vi "Read Spectra from Data Object.vi"(8 "error in (no error)":errorcluster, 10 "component":T1=32 items=["Magnitude^2"=37, "Magnitude"=32, "Phase"=33, "Real"=34, "Imaginary"=35, "Coherence"=36, "Unknown"=99], 11 "Y (1 Ch) in":refnum<class "Y (1 Ch).lvclass">) -> (0 "error out":errorcluster, 1 "spectra info":T2[](array[typedef]) {"x-axis units" items=["Time (s)"=0, "Frequency-CB (Hz)"=1, "Frequency-CPB (Hz)"=1248, "Frequency-Arbitrary (Hz)"=2357, "Quefrency (s)"=2, "Revolutions (rev)"=3, "Order"=4, "Speed (RPM)"=11, "Speed (rad/s)"=21, "Index"=65535]; "weighting filter" items=["Linear", "A-weighting", "B-weighting", "C-weighting", "ITU-R 468-4", "Dolby", "CCITT", "C-message", "Wb", "Wc", "Wd", "We", "Wf", "Wh", "Wj", "Wk", "Wm", "AES17 20 kHz lowpass", "AES17 40 kHz lowpass", "AES17 20 kHz highpass", "AES17 40 kHz highpass"]; "dB reference [EU]" format="%.2f"; "engineering units" items=["custom..."=0, "V"=1, "A"=21, "C"=30, "pC"=31, "s"=32, "-"=29, "Pa"=2, "N"=20, "g"=3, "m/s^2"=4, "m/s"=5, "m"=6, "mm/s"=12, "mm"=13, "micron/s"=14, "micron"=15, "in/s^2"=7, "in/s"=8, "in"=9, "mil/s"=10, "mil"=11, "rad/s^2"=16, "rad/s"=17, "rad"=18, "deg/s^2"=26, "deg/s"=27, "deg"=28, "RPM"=22, "cycle/s^2"=23, "Hz"=24, "cycle"=25, "strain"=19]; "spectral info"."window" items=["None "=0, "Hanning"=1, "Hamming"=2, "Blackman-Harris"=3, "Exact Blackman"=4, "Blackman"=5, "Flat Top"=6, "4 Term B-Harris "=7, "7 Term B-Harris"=8, "Low Sidelobe"=9, "Force - Exponential"=10, "Gaussian"=62]}, 2 "spectra":cluster{"x0":dbl, "dx":dbl, "Y":dbl[]}[](array[cluster]), 3 "Y (1 Ch) out":refnum<class "Y (1 Ch).lvclass">, 4 "global attributes":variant)   [LabVIEW 2017, in "Y (1 Ch).lvclass"]
uses:
  <vilib>/addons/_NISVFA/_Shared subVIs/Data Objects/Y (DBL)/Y (1 Ch).lvclass
  C:/Program Files (x86)/National Instruments/LabVIEW 2017/vi.lib/addons/_NISVFA/_Shared subVIs/Data Objects/Data/Data.lvclass
  <vilib>/addons/_NISVFA/_Shared subVIs/Controls/svc_Spectrum Info.ctl
  <vilib>/addons/_NISVFA/_Shared subVIs/Controls/svc_X-Axis Units.ctl
  <vilib>/addons/_NISVFA/_Shared subVIs/Controls/svc_Spectrum Type.ctl
  <vilib>/addons/_NISVFA/_Shared subVIs/Controls/svc_Engineering Units Text Ring.ctl
  <vilib>/addons/_NISVFA/_Shared subVIs/Controls/svc_Weighting Filter Text Ring.ctl
  <vilib>/addons/_NISVFA/_Shared subVIs/Controls/svc_Complimentary Spectrum Units.ctl
  <vilib>/addons/_NISVFA/_Shared subVIs/Controls/NI Spectrum Component.ctl
  <vilib>/addons/_NISVFA/_Shared subVIs/Data Objects/Data/Data.lvclass/Data.ctl
  <vilib>/addons/_NISVFA/_Shared subVIs/Common/sv_Get NI Property Name String.vi
  <vilib>/addons/_NISVFA/_Shared subVIs/Common/sv_Get SV Property Name String.vi
  <vilib>/addons/_NISVFA/_Shared subVIs/Common/svc_Spectrum Units.vi
  <vilib>/addons/_NISVFA/_Shared subVIs/Spectrum Info/sfva_Set SV Info in Spectrum Info Description.vi
  <vilib>/addons/_NISVFA/_Shared subVIs/Common/svc_Get Weighting Enum and Labels.vi
  <vilib>/addons/_NISVFA/_Shared subVIs/Common/svc_Unit Label Lexical Class.vi
  <vilib>/addons/_NISVFA/_Shared subVIs/Common/svc_Engineering Units to Unit Label.vi
  <vilib>/addons/_NISVFA/_Shared subVIs/Common/svc_Format Value (DBL).vi
  <vilib>/addons/_NISVFA/_Shared subVIs/Data Objects/Data/Data.lvclass
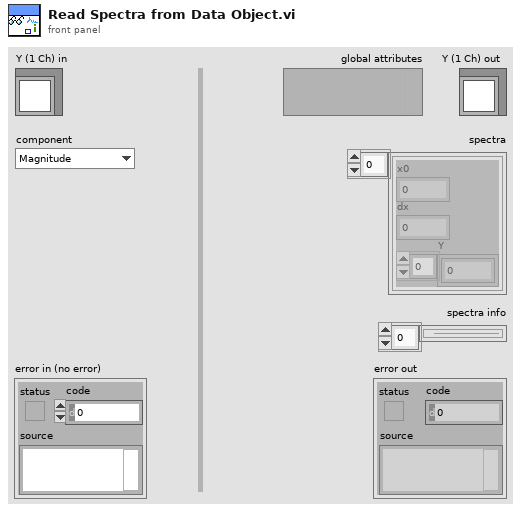
[diagram p1: front panel]
types:
  T1 = typedef "NI Spectrum Component.ctl" = u16
  T2 = typedef "svc_Spectrum Info.ctl" = cluster{"channel name":string, "description":string, "x-axis units":T3, "spectral info":cluster{"spectrum type":T4, "linear/dB":enum16{"linear", "dB"}, "window":u16, "window size":i32, "FFT size":i32}, "engineering units":T5, "custom label":string, "dB reference [EU]":dbl, "peak units":enum16{"rms", "peak", "peak-peak"}, "weighting filter":T6, "spectral density?":bool, "unit label":string, "spectrum skewed?":bool, "complimentary spectrum units":T7}
  T3 = typedef "svc_X-Axis Units.ctl" = u16
  T4 = typedef "svc_Spectrum Type.ctl" = enum16{"FFT Spectrum [complex]", "Amplitude [Magnitude]", "Power [Magnitude^2]", "Cross Spectrum [complex]", "Frequency Response [Complex]"}
  T5 = typedef "svc_Engineering Units Text Ring.ctl" = u16
  T6 = typedef "svc_Weighting Filter Text Ring.ctl" = u16
  T7 = typedef "svc_Complimentary Spectrum Units.ctl" = enum16{"none", "radians", "degrees", "cycles", "imaginary"}
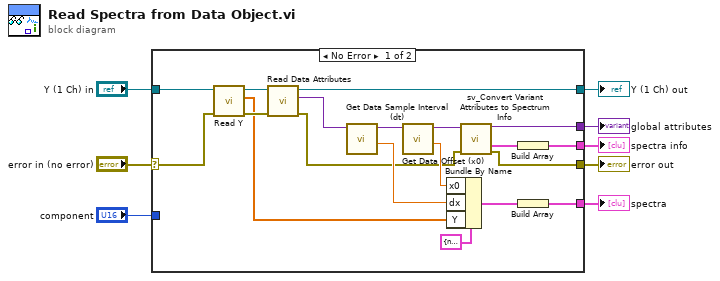
[diagram p0: block diagram]
diagram:
  n1 = case shown="No Error" "error in (no error)" {
    selector: "error in (no error)" -> [w11 w29]
    tunnel: [w9 w29] -> w7
    tunnel: [w19 w28] -> w5
    tunnel: "Y (1 Ch) in" -> [w20 w28]
    tunnel: [w22 _] -> w4
    tunnel: [w14 _] -> w3
    tunnel: [w12 _] -> w2
    tunnel: "component" -> [_ _]
    frame No Error {
      n2 = call <vilib>:"Read Y.vi"("error in (no error)"=w11, "Y (1Ch) in"=w20) -> ("error out"=w27:errorcluster, "Y"=w21:dbl[], "Y (1Ch) out"=w26:refnum<class "Y (1 Ch).lvclass">)  [unwired: 7 in]
      n3 = call <vilib>:"Read Data Attributes.vi"("error in (no error)"=w27, "Data in"=w26) -> ("error out"=w10:errorcluster, "data attributes"=w24:variant, "Data out"=w19:refnum<class "Y (1 Ch).lvclass">)  [unwired: 7 in]
      n4 = call <vilib>:"Get Data Sample Interval (dt).vi"("variant in"=w24) -> ("dt [s]"=w17:dbl, "variant out"=w25:variant)  [unwired: 9 in]
      n5 = call <vilib>:"Get Data Offset (x0).vi"("data attributes"=w25) -> ("x0"=w18:dbl, "data attributes"=w23:variant)  [unwired: 9 in]
      n6 = Bundle By Name(cluster=cluster{"x0":dbl, "dx":dbl, "Y":dbl[]} {"x0"=nan, "dx"=nan, "Y"=[nan]} ("power spectrum [dB EU]"), "x0"=w18, "dx"=w17, "Y"=w21) -> (w15:cluster{"x0":dbl, "dx":dbl, "Y":dbl[]})
      n7 = call <vilib>:"sv_Convert Variant Attributes to Spectrum Info.vi"("variant attributes"=w23, "error in"=w10) -> ("variant attributes"=w22:variant, "spectrum info"=w13:T2, "error out"=w9:errorcluster)  [unwired: 11 in]
      n8 = Build Array(w13) -> (w12:T2[])
      n9 = Build Array(w15) -> (w14:cluster{"x0":dbl, "dx":dbl, "Y":dbl[]}[])
    }
    frame Error {
    }
  }
  "error out" <- w7
  "Y (1 Ch) out" <- w5
  "global attributes" <- w4
  "spectra info" <- w2
  "spectra" <- w3
